vi "Teleop.vi"(10 "Match Info":T1={"Autonomous Elapsed Seconds"=0.0, "TeleOp Elapsed Seconds"=0.0, "Disabled Elapsed Seconds"=0.0, "Visited Autonomous"=FALSE, "Visited TeleOp"=FALSE, "Visited Disabled"=FALSE, "Autonomous Settings"={"Autonomous Style"=enum."Independent", "VI Refnum"=refnum}}, 11 "Call Context":T2) -> ()   [LabVIEW 2013]
doc: "This VI is called for each TeleOp packet received from the DS where the robot is not disabled. It is often used to read from the joysticks and update I/O or to update setpoints for timed control loops. It should complete and return within 20 milliseconds or it may miss DS packets."
uses:
  <vilib>/Rock Robotics/WPI/DriverStation/WPI_DriverStationDerivedRobotMode.ctl
  <vilib>/Rock Robotics/WPI/DriverStation/WPI_DriverStationMatch Info.ctl
  <vilib>/Rock Robotics/WPI/Solenoid/WPI_SolenoidValue.ctl
  Robot Global Data.vi
  <vilib>/Rock Robotics/WPI/Solenoid/Deprecated/WPI_SolenoidGetBool.vi
  <vilib>/Rock Robotics/WPI/Solenoid/WPI_SolenoidSetEnum.vi
  <vilib>/Rock Robotics/WPI/Joystick/WPI_JoystickGetSetRefNum.vi
  <vilib>/Rock Robotics/WPI/RobotDrive/WPI_RobotDriveGetSetRefNum.vi
panel:
  out "Ultrasoic Value":dbl
  out "Numeric 1":dbl(slide) scale=0.0..100.0
  out "Boolean 2":bool
  out "Boolean 1":bool
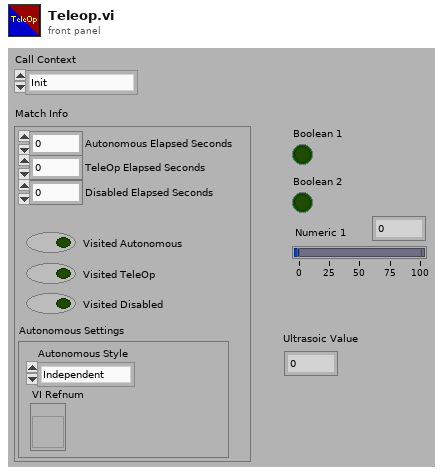
[diagram p1: front panel]
types:
  T1 = typedef "WPI_DriverStationMatch Info.ctl" = cluster{"Autonomous Elapsed Seconds":dbl, "TeleOp Elapsed Seconds":dbl, "Disabled Elapsed Seconds":dbl, "Visited Autonomous":bool, "Visited TeleOp":bool, "Visited Disabled":bool, "Autonomous Settings":cluster{"Autonomous Style":enum16{"Iterative", "Independent"}, "VI Refnum":refnum<vi>}}
  T2 = typedef "WPI_DriverStationDerivedRobotMode.ctl" = enum16{"Init", "Execute", "Stop"}
  T3 = typedef "WPI_JoystickDevRef.ctl" = cluster{"Device":T4}
  T4 = typedef "WPI_JoystickDeviceEnum.ctl" = enum16{"USB 1", "USB 2", "USB 3", "USB 4", "Kinect 1", "Kinect 2"}
  T5 = typedef "WPI_JoystickButtonState.ctl" = cluster{"Button 1":bool, "Button 2":bool, "Button 3":bool, "Button 4":bool, "Button 5":bool, "Button 6":bool, "Button 7":bool, "Button 8":bool, "Button 9":bool, "Button 10":bool, "Button 11":bool, "Button 12":bool}
  T6 = typedef "WPI_DigitalInputDevRef.ctl" = cluster{"DevStatus":errorcluster, "DIO Channel":T7, "Digital Module":T8}
  T7 = typedef "FPGA_DIOChannel.ctl" = enum8{"DIO 1", "DIO 2", "DIO 3", "DIO 4", "DIO 5", "DIO 6", "DIO 7", "DIO 8", "DIO 9", "DIO 10", "DIO 11", "DIO 12", "DIO 13", "DIO 14", "Invalid"}
  T8 = typedef "FPGA_TypedefDigitalModule.ctl" = enum16{"Digital Module 1", "Digital Module 2"}
  T9 = typedef "WPI_SolenoidDevRef.ctl" = cluster{"DevStatus":errorcluster, "Solenoid Module":T10, "Forward Solenoid Channel":T11, "Reverse Solenoid Channel":T11}
  T10 = typedef "FPGA_TypedefSolenoidModule.ctl" = enum16{"Solenoid Module 1", "Solenoid Module 2"}
  T11 = typedef "WPI_SolenoidChannel.ctl" = enum8{"Solenoid 1", "Solenoid 2", "Solenoid 3", "Solenoid 4", "Solenoid 5", "Solenoid 6", "Solenoid 7", "Solenoid 8", "Invalid"}
  T12 = typedef "WPI_RobotDriveDevRef.ctl" = cluster{"DevStatus":errorcluster, "Motors[]":T13[], "Square Inputs":bool, "Max Output":dbl, "Isochronous":bool}
  T13 = typedef "WPI_MotorControlDeviceRef.ctl" = cluster{"DeviceStatus":errorcluster, "Type":enum16{"PWM", "CAN"}, "PWM":cluster{"Digital Module":T8, "PWM Channel":T14, "DeadBand":T15}, "CAN":cluster{"Device Number":u8, "Control Mode":T16, "Semaphore":T17, "Max Vout":dbl}, "Invert":bool, "TransformRef":T18, "InvTransformRef":T18}
  T14 = typedef "FPGA_DIOPWMChannel.ctl" = enum8{"PWM 1", "PWM 2", "PWM 3", "PWM 4", "PWM 5", "PWM 6", "PWM 7", "PWM 8", "PWM 9", "PWM 10", "Invalid"}
  T15 = typedef "WPI_PWMDeadband.ctl" = cluster{"Name":string, "maxPositivePwm":i32, "minPositivePwm":i32, "centerPwm":i32, "maxNegativePwm":i32, "minNegativePwm":i32, "angularRange":u16}
  T16 = typedef "WPI_CANJaguar_ControlMode.ctl" = enum8{"Percent VBus", "Current", "Speed", "Position", "Voltage"}
  T17 = typedef "Semaphore RefNum" = refnum<k1>
  T18 = typedef "WPI_PWMTransform_ConPane.ctl" = refnum<vi>
  T19 = cluster{"axis 1 (x)":dbl, "axis 2 (y)":dbl, "axis 3 (throttle)":dbl, "axis 4":dbl, "axis 5":dbl, "axis 6":dbl}
  T20 = typedef "WPI_SolenoidValue.ctl" = enum16{"Off", "On", "Forward", "Reverse"}
  T21 = typedef "WPI_AnalogChannelDevRef.ctl" = cluster{"DevStatus":errorcluster, "Analog Module":T22, "Analog Channel":T23}
  T22 = typedef "FPGA_TypedefAnalogModule.ctl" = enum16{"Analog Module 1", "Analog Module 2"}
  T23 = typedef "FPGA_AIChannel.ctl" = enum8{"AI 1", "AI 2", "AI 3", "AI 4", "AI 5", "AI 6", "AI 7", "AI 8", "Invalid"}
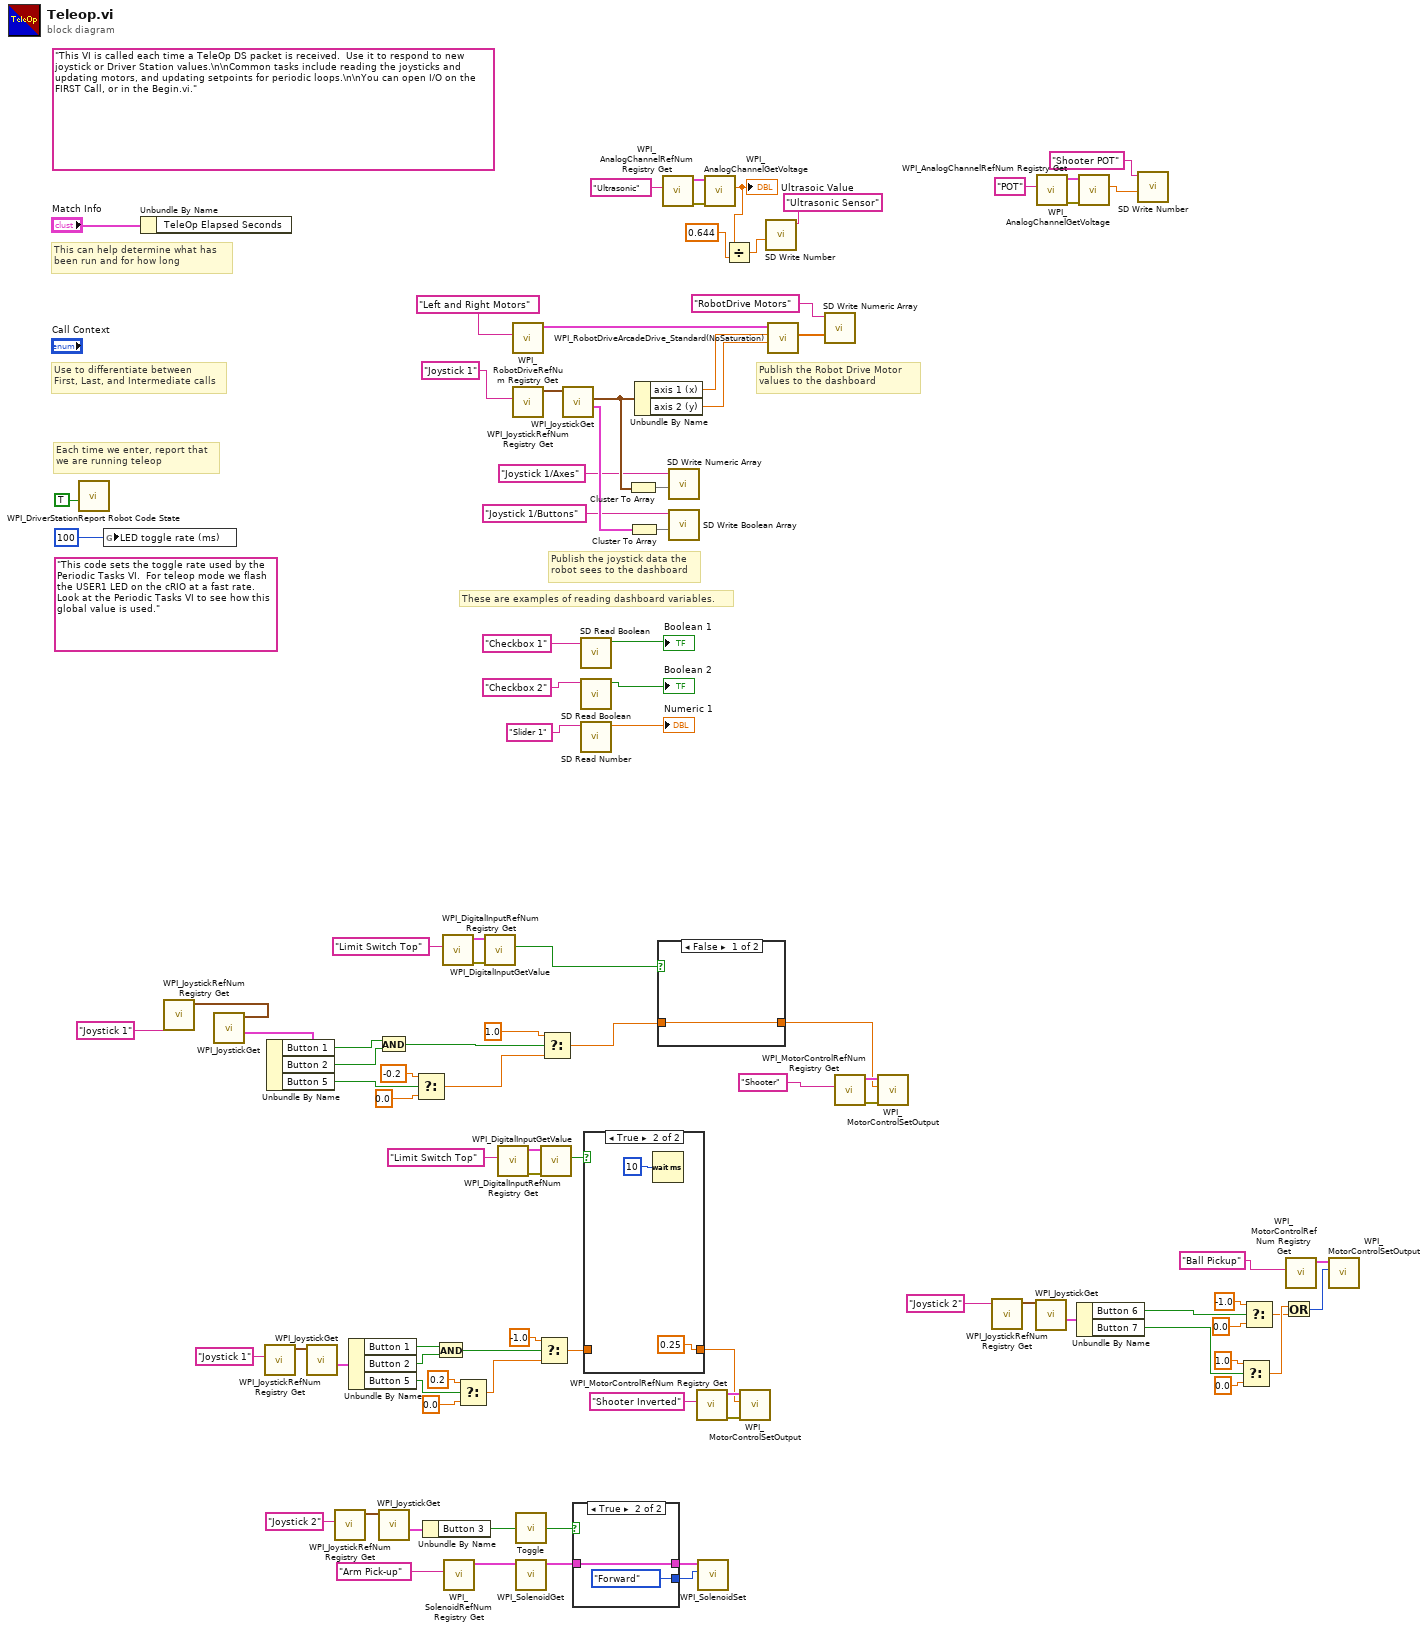
[diagram p0: block diagram]
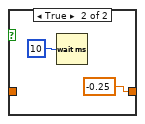
[diagram p3: hidden frame]
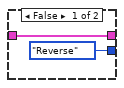
[diagram p4: hidden frame]
diagram:
  (unwired) "This code sets the toggle rate used by the Periodic Tasks VI.  For teleop mode we flash the USER1 LED on the cRIO at a fast rate.  Look at the Periodic Tasks VI to see how this global value is used."
  (unwired) "This VI is called each time a TeleOp DS packet is received.  Use it to respond to new joystick or Driver Station values.\n\nCommon tasks include reading the joysticks and updating motors, and updating setpoints for periodic loops.\n\nYou can open I/O on the FIRST Call, or in the Begin.vi."
  # "These are examples of reading dashboard variables."
  # "Publish the Robot Drive Motor\nvalues to the dashboard"
  # "Publish the joystick data the\nrobot sees to the dashboard"
  # "Each time we enter, report that\nwe are running teleop"
  # "Use to differentiate between\nFirst, Last, and Intermediate calls"
  # "This can help determine what has\nbeen run and for how long"
  n1 = call <vilib>:"WPI_DriverStationReport Robot Code State.vi"("TeleOp"=TRUE ("Autonomous")) -> ()  [unwired: 10 in, 1 out]
  n2 = global write "Robot Global Data.vi" "LED toggle rate (ms)"(u32 100 ("LED ms toggle rate")) -> ()
  n3 = Unbundle By Name("Match Info") -> ()  [unwired: 1 out]
  n4 = call <vilib>:"WPI_JoystickRefNum Registry Get.vi"("refnum name"="Joystick 1") -> ("JoystickDevRef"=w75:T3)  [unwired: 9 in, 1 out]
  n5 = call <vilib>:"WPI_JoystickGet.vi"("JoystickDevRef"=w75) -> ("Buttons"=w74:T5)  [unwired: 4 in, 2 out]
  n6 = call <vilib>:"WPI_JoystickRefNum Registry Get.vi"("refnum name"="Joystick 1") -> ("JoystickDevRef"=w68:T3)  [unwired: 9 in, 1 out]
  n7 = Unbundle By Name(w74) -> ("Button 1"=w18:bool, "Button 2"=w17:bool, "Button 5"=w15:bool)
  n8 = call <vilib>:"WPI_JoystickGet.vi"("JoystickDevRef"=w68) -> ("Buttons"=w69:T5)  [unwired: 4 in, 2 out]
  n9 = call <vilib>:"WPI_JoystickRefNum Registry Get.vi"("refnum name"="Joystick 2") -> ("JoystickDevRef"=w50:T3)  [unwired: 9 in, 1 out]
  n10 = Unbundle By Name(w69) -> ("Button 1"=w19:bool, "Button 2"=w20:bool, "Button 5"=w16:bool)
  n11 = And(x=w18, y=w17) -> (x .and. y?=w43:bool)
  n12 = call <vilib>:"WPI_JoystickGet.vi"("JoystickDevRef"=w50) -> ("Buttons"=w49:T5)  [unwired: 4 in, 2 out]
  n13 = Select(t=-0.2, s=w15, f=0.0) -> (s? t:f=w22:dbl)
  n14 = Unbundle By Name(w49) -> ("Button 3"=w29:bool)
  n15 = And(x=w19, y=w20) -> (x .and. y?=w70:bool)
  n16 = call <vilib>:"WPI_DigitalInputRefNum Registry Get.vi"("refnum name"="Limit Switch Top") -> ("error out"=w41:errorcluster, "DigitalInputDevRef"=w40:T6)  [unwired: 9 in]
  n17 = call <vilib>:"WPI_SolenoidRefNum Registry Get.vi"("refnum name"="Arm Pick-up") -> ("SolenoidDevRef"=w48:T9)  [unwired: 9 in, 1 out]
  n18 = Select(t=0.2, s=w16, f=0.0) -> (s? t:f=w21:dbl)
  n19 = call <vilib>:"WPI_DigitalInputGetValue.vi"("error in (no error)"=w41, "DigitalInputDevRef"=w40) -> ("Value"=w39:bool)  [unwired: 7 in, 2 out]
  n20 = call <vilib>:"WPI_DigitalInputRefNum Registry Get.vi"("refnum name"="Limit Switch Top") -> ("error out"=w36:errorcluster, "DigitalInputDevRef"=w37:T6)  [unwired: 9 in]
  n21 = call <vilib>:"WPI_RobotDriveRefNum Registry Get.vi"("refnum name"="Left and Right Motors") -> ("RobotDriveDevRef"=w97:T12)  [unwired: 1 in, 9 out]
  n22 = call <vilib>:"WPI_JoystickRefNum Registry Get.vi"("refnum name"="Joystick 1") -> ("JoystickDevRef"=w93:T3)  [unwired: 1 in, 9 out]
  n23 = call "Toggle.vi"("Input"=w29) -> ("Toggled Output"=w47:bool)
  n24 = call-poly <vilib>:"WPI_SolenoidGet.vi"("SolenoidDevRef"=w48) -> ("SolenoidDevRef"=w46:T9)  [unwired: 8 in, 2 out]
  n25 = Select(t=-1.0, s=w70, f=w21) -> (s? t:f=w33:dbl)
  n26 = call <vilib>:"WPI_DigitalInputGetValue.vi"("error in (no error)"=w36, "DigitalInputDevRef"=w37) -> ("Value"=w34:bool)  [unwired: 7 in, 2 out]
  n27 = Select(t=1.0, s=w43, f=w22) -> (s? t:f=w38:dbl)
  n28 = call <vilib>:"WPI_JoystickGet.vi"("JoystickDevRef"=w93) -> ("Buttons"=w90:T5, "Axes"=w87:T19)  [unwired: 1 in, 4 out]
  n29 = case shown="True" w47 {
    tunnel: w46 -> [w101 w103]
    tunnel: [w101 w103] -> w45
    tunnel: [WPI_SolenoidValue."Reverse" ("Value") WPI_SolenoidValue."Forward" ("Value")] -> w44
    frame False {
    }
    frame True {
    }
  }
  n30 = call <vilib>:"SD Read Boolean.vi"("Name"="Checkbox 1" ("refnum name")) -> ("Boolean"=→"Boolean 1":bool)  [unwired: 8 in, 2 out]
  n31 = call <vilib>:"SD Read Boolean.vi"("Name"="Checkbox 2" ("refnum name")) -> ("Boolean"=→"Boolean 2":bool)  [unwired: 8 in, 2 out]
  n32 = call <vilib>:"SD Read Number.vi"("Name"="Slider 1" ("refnum name")) -> ("Numeric"=→"Numeric 1":dbl)  [unwired: 8 in, 2 out]
  n33 = case shown="True" w34 {
    tunnel: [w104 0.25 ("f")] -> w10
    tunnel: w33 -> [w104 _]
    frame False {
    }
    frame True {
      n34 = Wait (ms)(milliseconds to wait=u32 10) -> ()  [unwired: 1 out]
    }
  }
  n35 = Cluster To Array(cluster=w87) -> (array=w86:dbl[])
  n36 = Cluster To Array(cluster=w90) -> (array=w89:bool[])
  n37 = Unbundle By Name(w87) -> ("axis 1 (x)"=w96:dbl, "axis 2 (y)"=w95:dbl)
  n38 = case shown="False" w39 {
    tunnel: [w107 -0.25 ("f")] -> w11
    tunnel: w38 -> [w107 _]
    frame False {
    }
    frame True {
      n39 = Wait (ms)(milliseconds to wait=u32 10) -> ()  [unwired: 1 out]
    }
  }
  n40 = call <vilib>:"WPI_AnalogChannelRefNum Registry Get.vi"("refnum name"="Ultrasonic") -> ("error out"=w31:errorcluster, "AIDeviceRef"=w30:T21)  [unwired: 9 in]
  n41 = call <vilib>:"SD Write Numeric Array.vi"("Numeric Array"=w86, "Name"="Joystick 1/Axes") -> ()  [unwired: 8 in, 2 out]
  n42 = call <vilib>:"SD Write Boolean Array.vi"("Boolean Array"=w89, "Name"="Joystick 1/Buttons") -> ()  [unwired: 8 in, 2 out]
  n43 = call <vilib>:"WPI_MotorControlRefNum Registry Get.vi"("refnum name"="Shooter Inverted") -> ("error out"=w13:errorcluster, "MotorControlDevRef"=w14:T13)  [unwired: 9 in]
  n44 = call-poly <vilib>:"WPI_SolenoidSet.vi"("Value"=w44, "SolenoidDevRef"=w45) -> ()  [unwired: 8 in, 2 out]
  n45 = call <vilib>:"WPI_AnalogChannelGetVoltage.vi"("error in (no error)"=w31, "AIDeviceRef"=w30) -> ("Voltage"=w7:dbl)  [unwired: 7 in, 2 out]
  "Ultrasoic Value" <- w7
  n46 = Divide(x=w7, y=0.644) -> (x/y=w6:dbl)
  n47 = call <vilib>:"WPI_MotorControlSetOutput.vi"("error in (no error)"=w13, "Output"=w10, "MotorControlDevRef"=w14) -> ()  [unwired: 6 in, 3 out]
  n48 = call <vilib>:"SD Write Number.vi"("Numeric"=w6, "Name"="Ultrasonic Sensor") -> ()  [unwired: 8 in, 2 out]
  n49 = call <vilib>:"WPI_RobotDriveArcadeDrive_Standard(NoSaturation).vi"("Y axis value"=w95, "X axis value"=w96, "RobotDriveDevRef"=w97) -> ("Motor Values"=w83:dbl[])  [unwired: 1 in, 7 out]
  n50 = call <vilib>:"SD Write Numeric Array.vi"("Numeric Array"=w83, "Name"="RobotDrive Motors") -> ()  [unwired: 8 in, 2 out]
  n51 = call <vilib>:"WPI_MotorControlRefNum Registry Get.vi"("refnum name"="Shooter") -> ("error out"=w72:errorcluster, "MotorControlDevRef"=w71:T13)  [unwired: 9 in]
  n52 = call <vilib>:"WPI_MotorControlSetOutput.vi"("error in (no error)"=w72, "Output"=w11, "MotorControlDevRef"=w71) -> ()  [unwired: 6 in, 3 out]
  n53 = call <vilib>:"WPI_JoystickRefNum Registry Get.vi"("refnum name"="Joystick 2") -> ("JoystickDevRef"=w58:T3)  [unwired: 9 in, 1 out]
  n54 = call <vilib>:"WPI_JoystickGet.vi"("JoystickDevRef"=w58) -> ("Buttons"=w59:T5)  [unwired: 4 in, 2 out]
  n55 = call <vilib>:"WPI_AnalogChannelRefNum Registry Get.vi"("refnum name"="POT") -> ("error out"=w4:errorcluster, "AIDeviceRef"=w5:T21)  [unwired: 9 in]
  n56 = Unbundle By Name(w59) -> ("Button 6"=w60:bool, "Button 7"=w56:bool)
  n57 = call <vilib>:"WPI_AnalogChannelGetVoltage.vi"("error in (no error)"=w4, "AIDeviceRef"=w5) -> ("Voltage"=w2:dbl)  [unwired: 7 in, 2 out]
  n58 = call <vilib>:"SD Write Number.vi"("Numeric"=w2, "Name"="Shooter POT" ("Table Prefix out")) -> ()  [unwired: 8 in, 2 out]
  n59 = Select(t=1.0, s=w56, f=0.0) -> (s? t:f=w55:dbl)
  n60 = Select(t=-1.0, s=w60, f=0.0) -> (s? t:f=w54:dbl)
  n61 = Or(x=w55, y=w54) -> (x .or. y?=w53:i32)
  n62 = call <vilib>:"WPI_MotorControlRefNum Registry Get.vi"("refnum name"="Ball Pickup") -> ("MotorControlDevRef"=w65:T13)  [unwired: 9 in, 1 out]
  n63 = call <vilib>:"WPI_MotorControlSetOutput.vi"("Output"=w53, "MotorControlDevRef"=w65) -> ()  [unwired: 7 in, 3 out]
